vi "Write make lower case (F).vi"(8 "error in (no error)":errorcluster, 10 "make lower case (F)":bool, 11 "control label adjustment in":refnum<class "control label adjustment.lvclass">) -> (0 "error out":errorcluster, 3 "control label adjustment out":refnum<class "control label adjustment.lvclass">)   [LabVIEW 2013, in "control label adjustment.lvclass"]
uses:
  control label adjustment.lvclass
  control label adjustment.lvclass/control label adjustment.ctl
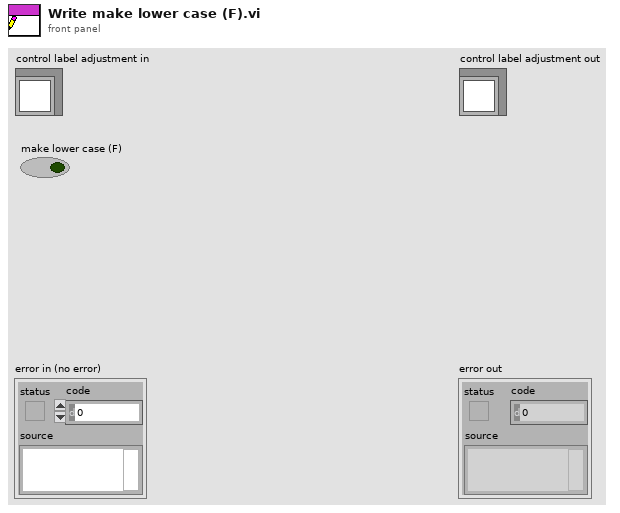
[diagram p1: front panel]
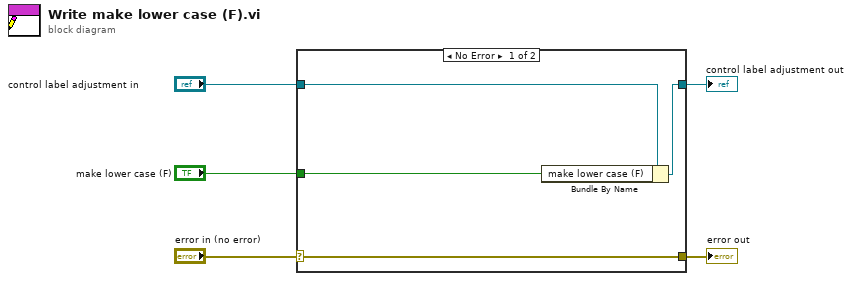
[diagram p0: block diagram]
diagram:
  n1 = case shown="No Error" "error in (no error)" {
    selector: "error in (no error)" -> [w9 w10]
    tunnel: [w9 w10] -> w4
    tunnel: [w7 w11] -> w2
    tunnel: "control label adjustment in" -> [w8 w11]
    tunnel: "make lower case (F)" -> [w6 _]
    frame No Error {
      n2 = Bundle By Name(cluster=w8, "make lower case (F)"=w6) -> (w7:refnum<class "control label adjustment.lvclass">)
    }
    frame Error {
    }
  }
  "error out" <- w4
  "control label adjustment out" <- w2
